vi "CLD 13 Timer w flow sensitivity.vi"(8 "Error In":errorcluster, 10 "Flow Rate":i8(slide) min=-2 max=2 step=1 scale=-2.0..2.0, 11 "Timer Enum":T1) -> (0 "Error Out":errorcluster, 3 "Time elapsed":dbl)   [LabVIEW 2018]
doc: "CLD 13 This timer will reset itself when the input flow rate is zero."
uses:
  CLD 13 timer Enum.ctl
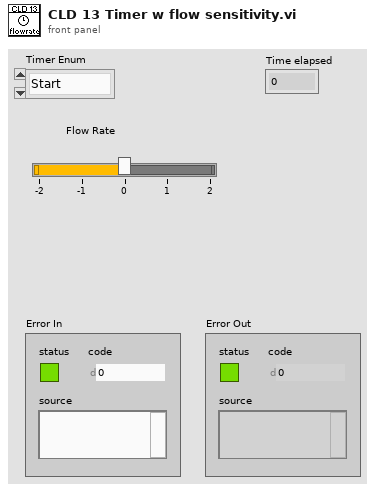
[diagram p1: front panel]
types:
  T1 = typedef "CLD 13 timer Enum.ctl" = enum16{"Start", "Read"}
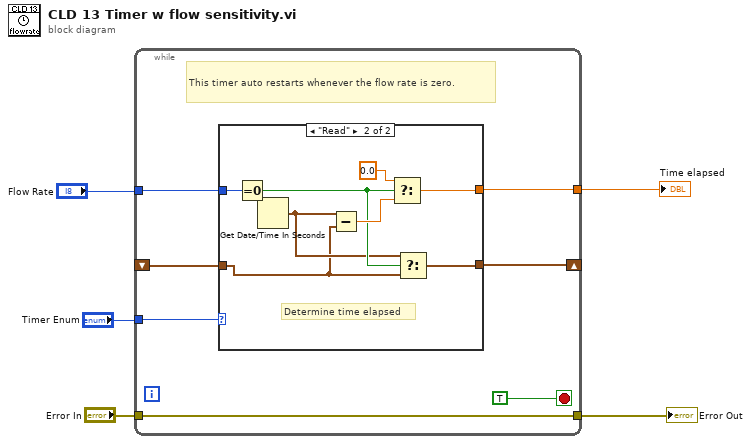
[diagram p0: block diagram]
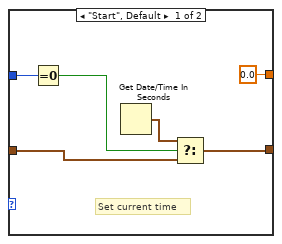
[diagram p2: hidden frame]
diagram:
  n1 = while {
    tunnel: "Timer Enum" -> [w11]
    shift-right: [w10] -> _
    shift-left: _ -> [w9]
    tunnel: [w8] -> w4
    tunnel: "Flow Rate" -> [w7]
    tunnel: [w6] -> w1
    tunnel: "Error In" -> [w6]
    stop <- TRUE stop-if-true
    # "This timer auto restarts whenever the flow rate is zero."
    n2 = case shown="\"Read\"" w11 {
      tunnel: [w14 w19] -> w10
      tunnel: w9 -> [w13 w20]
      tunnel: [0.0 w25] -> w8
      tunnel: w7 -> [w17 w23]
      frame "Start", Default {
        # "Set current time"
        n3 = Equal To 0?(x=w17) -> (x = 0?=w16:bool)
        n4 = Get Date/Time In Seconds() -> (seconds since 1Jan1904=w15:timestamp)
        n5 = Select(t=w15, s=w16, f=w13) -> (s? t:f=w14:timestamp)
      }
      frame "Read" {
        # "Determine time elapsed"
        n6 = Equal To 0?(x=w23) -> (x = 0?=w22:bool)
        n7 = Get Date/Time In Seconds() -> (seconds since 1Jan1904=w21:timestamp)
        n8 = Subtract(x=w21, y=w20) -> (x-y=w26:dbl)
        n9 = Select(t=0.0, s=w22, f=w26) -> (s? t:f=w25:dbl)
        n10 = Select(t=w21, s=w22, f=w20) -> (s? t:f=w19:timestamp)
      }
    }
  }
  "Time elapsed" <- w4
  "Error Out" <- w1
